vi "Get Oldest Time to Plot.vi"(8 "reset? [F]":bool, 9 "History Length (s)":dbl=1800.0 format="%<%M:%S>t", 11 "Clear Plot [F]":bool) -> (1 "clear button active?":bool, 3 "Oldest Time to Plot":u64)   [LabVIEW 2021, in "RocketPlot.lvlib"]
uses:
  RocketPlot.lvlib
  d285c313-a79c-4602-b75e-186d55f373a0.vi
  c791649b-4a78-4eca-b450-b650c181913e.vi
  <userlib>/bjustice/Ring Buffer for Time Series Data Strict Accessor/Unix time epoch/Unix_Epoch_in_Labview.vi
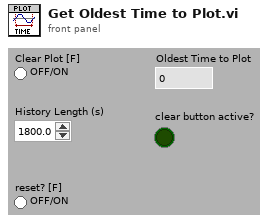
[diagram p1: front panel]
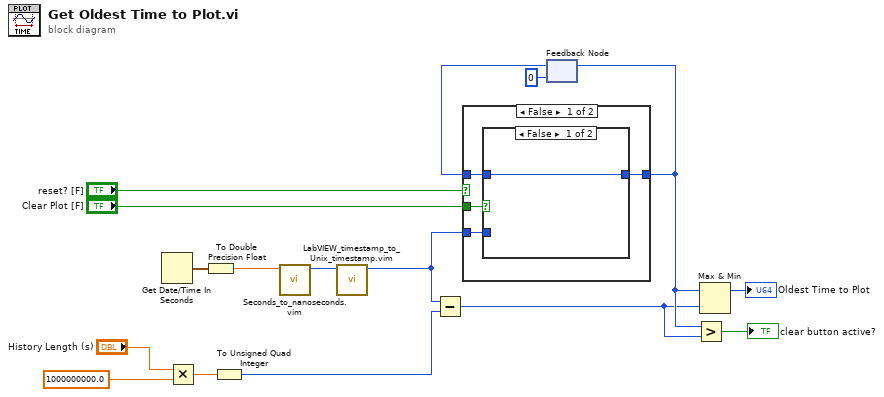
[diagram p0: block diagram]
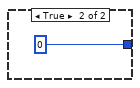
[diagram p3: hidden frame]
diagram:
  n1 = Get Date/Time In Seconds() -> (seconds since 1Jan1904=w4:timestamp)
  n2 = Multiply(x="History Length (s)", y=1000000000.0) -> (x*y=w6:dbl)
  n3 = To Double Precision Float(number=w4) -> (double precision float=w2:dbl)
  n4 = To Unsigned Quad Integer(1:w6) -> (0:w5:u64)
  n5 = call "Seconds_to_nanoseconds.vim"("timestamp (seconds)"=w2) -> ("timestamp (nanoseconds)"=w3:u64)  [unwired: 10 in]
  n6 = call "LabVIEW_timestamp_to_Unix_timestamp.vim"("LabVIEW timestamp (nanoseconds)"=w3) -> ("Unix timestamp (nanoseconds)"=w1:u64)  [unwired: 10 in]
  n7 = Subtract(x=w1, y=w5) -> (x-y=w10:u64)
  n8 = feedback #1(u64 0) -> (w12:u64)
  n9 = case shown="False" "reset? [F]" {
    tunnel: [w18 u64 0] -> w11
    tunnel: "Clear Plot [F]" -> [w20 _]
    tunnel: w1 -> [w19 _]
    tunnel: w12 -> [w17 _]
    frame False {
      n10 = case shown="False" w20 {
        tunnel: w19 -> [_ w22]
        tunnel: [w21 w22] -> w18
        tunnel: w17 -> [w21 _]
        frame False {
        }
        frame True {
        }
      }
    }
    frame True {
    }
  }
  n11 = feedback-in #1(w11) -> ()
  n12 = Greater?(x=w11, y=w10) -> (0:→"clear button active?":bool)
  n13 = Max & Min(x=w11, y=w10) -> (max(x,y)=→"Oldest Time to Plot":u64)  [unwired: 1 out]
